vi "Capitalize String.vi"(11 "String":string) -> (3 "Capitalized String":string)   [LabVIEW 2014]
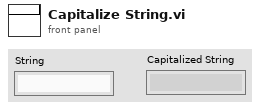
[diagram p1: front panel]
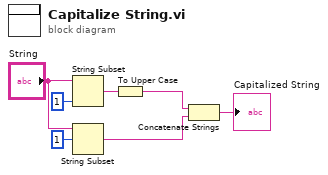
[diagram p0: block diagram]
diagram:
  n1 = String Subset(string="String", length (rest)=1 ("length (rest)")) -> (substring=w4:string)  [unwired: 1 in]
  n2 = String Subset(string="String", offset (0)=1) -> (substring=w2:string)  [unwired: 1 in]
  n3 = To Upper Case(1:w4) -> (0:w3:string)
  n4 = Concatenate Strings(w3, w2) -> (→"Capitalized String":string)
